vi "RPL_top_level_GUI_2.vi"() -> ()   [LabVIEW 2021]
uses:
  <vilib>/Utility/file.llb/Read Delimited Spreadsheet (string).vi
panel:
  out "Abort Status":string
  out "sol2":bool[](array[boolean])
  in  "Time Target (s)":dbl=1.0
  out "Array":string[][](array[string])
  in  "?":bool
  in  "Absolute Change":dbl
  out "ABORT\nACTIVATED":bool
  out "% Change":dbl[](array[numeric])
  in  "% Change":dbl
  out "all rows":string[][](array[string])
  in  "Fire Button":bool
  out "IGNITION":bool
  out "DEADMAN\nSWITCH":bool
  in  "Arm Button":bool
  out "POWER DISCONNECTED":bool
  in  "?":bool
  in  "SV6":bool
  in  "SV5":bool
  in  "SV4":bool
  in  "?":bool
  in  "SV3":bool
  in  "SV2":bool
  in  "SV1":bool
  in  "SV0":bool
  in  "GUITabs":T1(tab) caption="Tab Control"
  in  "Deadman Switch Pin":u16(ring) items=["FIO0", "FIO1", "FIO2", "FIO3", "FIO4", "FIO5", "FIO6", "FIO7", "EIO0", "EIO1", "EIO2", "EIO3", "EIO4", "EIO5", "EIO6", "EIO7", "CIO0", "CIO1", "CIO2", "CIO3", "MIO0", "MIO1", "MIO2"]
  in  "Solenoid Supply Pin":u16=5
  in  "LabJack Supply Pin":u16=7
  in  "Relay Supply Pin":u16=9
  in  "Igniter Pin":u16(ring)=7 items=["FIO0", "FIO1", "FIO2", "FIO3", "FIO4", "FIO5", "FIO6", "FIO7", "EIO0", "EIO1", "EIO2", "EIO3", "EIO4", "EIO5", "EIO6", "EIO7", "CIO0", "CIO1", "CIO2", "CIO3", "MIO0", "MIO1", "MIO2"]
  in  "LabJack IP Address":string="192.168.1.199"
  in  "LabJack Connection Type":u16(ring) items=["USB", "Ethernet"]
  in  "S: NO/NC":bool=TRUE
  in  "SV0 Pin":u16(ring)=8 items=["FIO0", "FIO1", "FIO2", "FIO3", "FIO4", "FIO5", "FIO6", "FIO7", "EIO0", "EIO1", "EIO2", "EIO3", "EIO4", "EIO5", "EIO6", "EIO7", "CIO0", "CIO1", "CIO2", "CIO3", "MIO0", "MIO1", "MIO2"]
  in  "SV1 Pin":u16(ring)=9 items=["FIO0", "FIO1", "FIO2", "FIO3", "FIO4", "FIO5", "FIO6", "FIO7", "EIO0", "EIO1", "EIO2", "EIO3", "EIO4", "EIO5", "EIO6", "EIO7", "CIO0", "CIO1", "CIO2", "CIO3", "MIO0", "MIO1", "MIO2"]
  in  "SV3 Pin":u16(ring)=11 items=["FIO0", "FIO1", "FIO2", "FIO3", "FIO4", "FIO5", "FIO6", "FIO7", "EIO0", "EIO1", "EIO2", "EIO3", "EIO4", "EIO5", "EIO6", "EIO7", "CIO0", "CIO1", "CIO2", "CIO3", "MIO0", "MIO1", "MIO2"]
  in  "SV2 Pin":u16(ring)=10 items=["FIO0", "FIO1", "FIO2", "FIO3", "FIO4", "FIO5", "FIO6", "FIO7", "EIO0", "EIO1", "EIO2", "EIO3", "EIO4", "EIO5", "EIO6", "EIO7", "CIO0", "CIO1", "CIO2", "CIO3", "MIO0", "MIO1", "MIO2"]
  in  "SV6 Pin":u16(ring)=14 items=["FIO0", "FIO1", "FIO2", "FIO3", "FIO4", "FIO5", "FIO6", "FIO7", "EIO0", "EIO1", "EIO2", "EIO3", "EIO4", "EIO5", "EIO6", "EIO7", "CIO0", "CIO1", "CIO2", "CIO3", "MIO0", "MIO1", "MIO2"]
  in  "SV5 Pin":u16(ring)=13 items=["FIO0", "FIO1", "FIO2", "FIO3", "FIO4", "FIO5", "FIO6", "FIO7", "EIO0", "EIO1", "EIO2", "EIO3", "EIO4", "EIO5", "EIO6", "EIO7", "CIO0", "CIO1", "CIO2", "CIO3", "MIO0", "MIO1", "MIO2"]
  in  "SV4 Pin":u16(ring)=12 items=["FIO0", "FIO1", "FIO2", "FIO3", "FIO4", "FIO5", "FIO6", "FIO7", "EIO0", "EIO1", "EIO2", "EIO3", "EIO4", "EIO5", "EIO6", "EIO7", "CIO0", "CIO1", "CIO2", "CIO3", "MIO0", "MIO1", "MIO2"]
  in  "S: NO/NC":bool=TRUE
  in  "S: NO/NC":bool=TRUE
  in  "S: NO/NC":bool=TRUE
  in  "S: NO/NC":bool=TRUE
  in  "S: NO/NC":bool=TRUE
  in  "S: NO/NC":bool=TRUE
  in  "R: NC/NO":bool=TRUE
  in  "R: NC/NO":bool=TRUE
  in  "R: NC/NO":bool=TRUE
  in  "R: NC/NO":bool=TRUE
  in  "R: NC/NO":bool=TRUE
  in  "R: NC/NO":bool=TRUE
  in  "R: NC/NO":bool=TRUE
  in  "TC1 Type":u16(ring)=7 items=["B", "E", "J", "K", "N", "R", "S", "T"]
  in  "TC2 Type":u16(ring)=3 items=["B", "E", "J", "K", "N", "R", "S", "T"]
  in  "TC1 +Channel":u16
  in  "TC2 -Channel":u16=3
  in  "TC2 +Channel":u16=2
  in  "TC1 -Channel":u16=1
  in  "PT2 Pin":u16=6
  in  "PT1 Pin":u16=8
  in  "PT3 Pin":u16=4
  in  "LP1 Pin":u16=10
  in  "k [N/m]":dbl=2000.0
  out "?":u32[](array[numeric])
  out "?":bool[](array[boolean])
  out "?":string[](array[string])
  in  "SV0":bool
  out "?":bool[](array[boolean])
  out "?":bool[](array[boolean])
  out "?":bool[](array[boolean])
  in  "SV1":bool
  in  "SV2":bool
  in  "SV3":bool
  out "?":bool[](array[boolean])
  in  "SV4":bool
  out "?":bool[](array[boolean])
  out "?":bool[](array[boolean])
  in  "SV5":bool
  in  "SV6":bool
  in  "Procedure Name":string
  in  "P#":u32
  in  "Add Procedure":bool
  in  "Remove Procedure":bool
  in  "Row":u32
  out "?":u32[](array[numeric])
  out "File Path":path[](array[path])
  out "?":bool
  out "?":bool
  out "?":bool
  out "?":bool
  out "?":bool
  out "?":bool
  out "?":bool
  out "?":bool
  out "?":bool
  out "?":bool
  out "?":bool
  out "?":bool
  out "?":bool
  in  "Dry Test-Run":bool
  out "LabJack Supply Voltage":dbl(slide) scale=0.0..5.0
  out "Solenoid Supply Voltage":dbl(slide) scale=0.0..14.0
  out "Relay Supply Voltage":dbl(slide) scale=0.0..5.0
  out "?":bool
  out "?":bool
  out "?":bool
  out "PT3: Chamber Pressure [psi]":dbl(knob) scale=0.0..500.0
  out "TC1: N2O Temp [°C]":dbl(slide) scale=-20.0..20.0
  out "TC2: Chamber Temp [°C]":dbl(slide) scale=-270.0..1260.0
  out "LP1: Thrust Reading [N]":dbl(slide) scale=0.0..250.0
  out "PT1: N2O Pressure [psi]":dbl(knob) scale=0.0..1000.0
  out "PT2: Ethanol Pressure [psi]":dbl(knob) scale=0.0..1000.0
  out "?":bool
  out "?":bool
  out "?":dbl[][](graph)
  in  "DATA LOGGING":bool
  in  "?":bool
  in  "?":bool
  # "SYSTEM FIRE OPERATION"
  # "CONTROL & ABORT STATUS"
  # "FEED SYSTEM SETTINGS"
  # "HIL TEST PARAMETERS"
  # "THERMOCOUPLE SETTINGS"
  # "SOLENOID VALVE & RELAY SETTINGS"
  # "CALIBRATION SETTINGS"
  # "POWER SYSTEM SETTINGS"
  # "THRUST MEASUREMENT SETTINGS"
  # "LINE & CHAMBER STATUS"
  # "RUNTANK FLOWRATE STATUS"
  # "DATA LOGGING"
  # "POWER SUPPLY STATUS"
  # "THRUST STATUS"
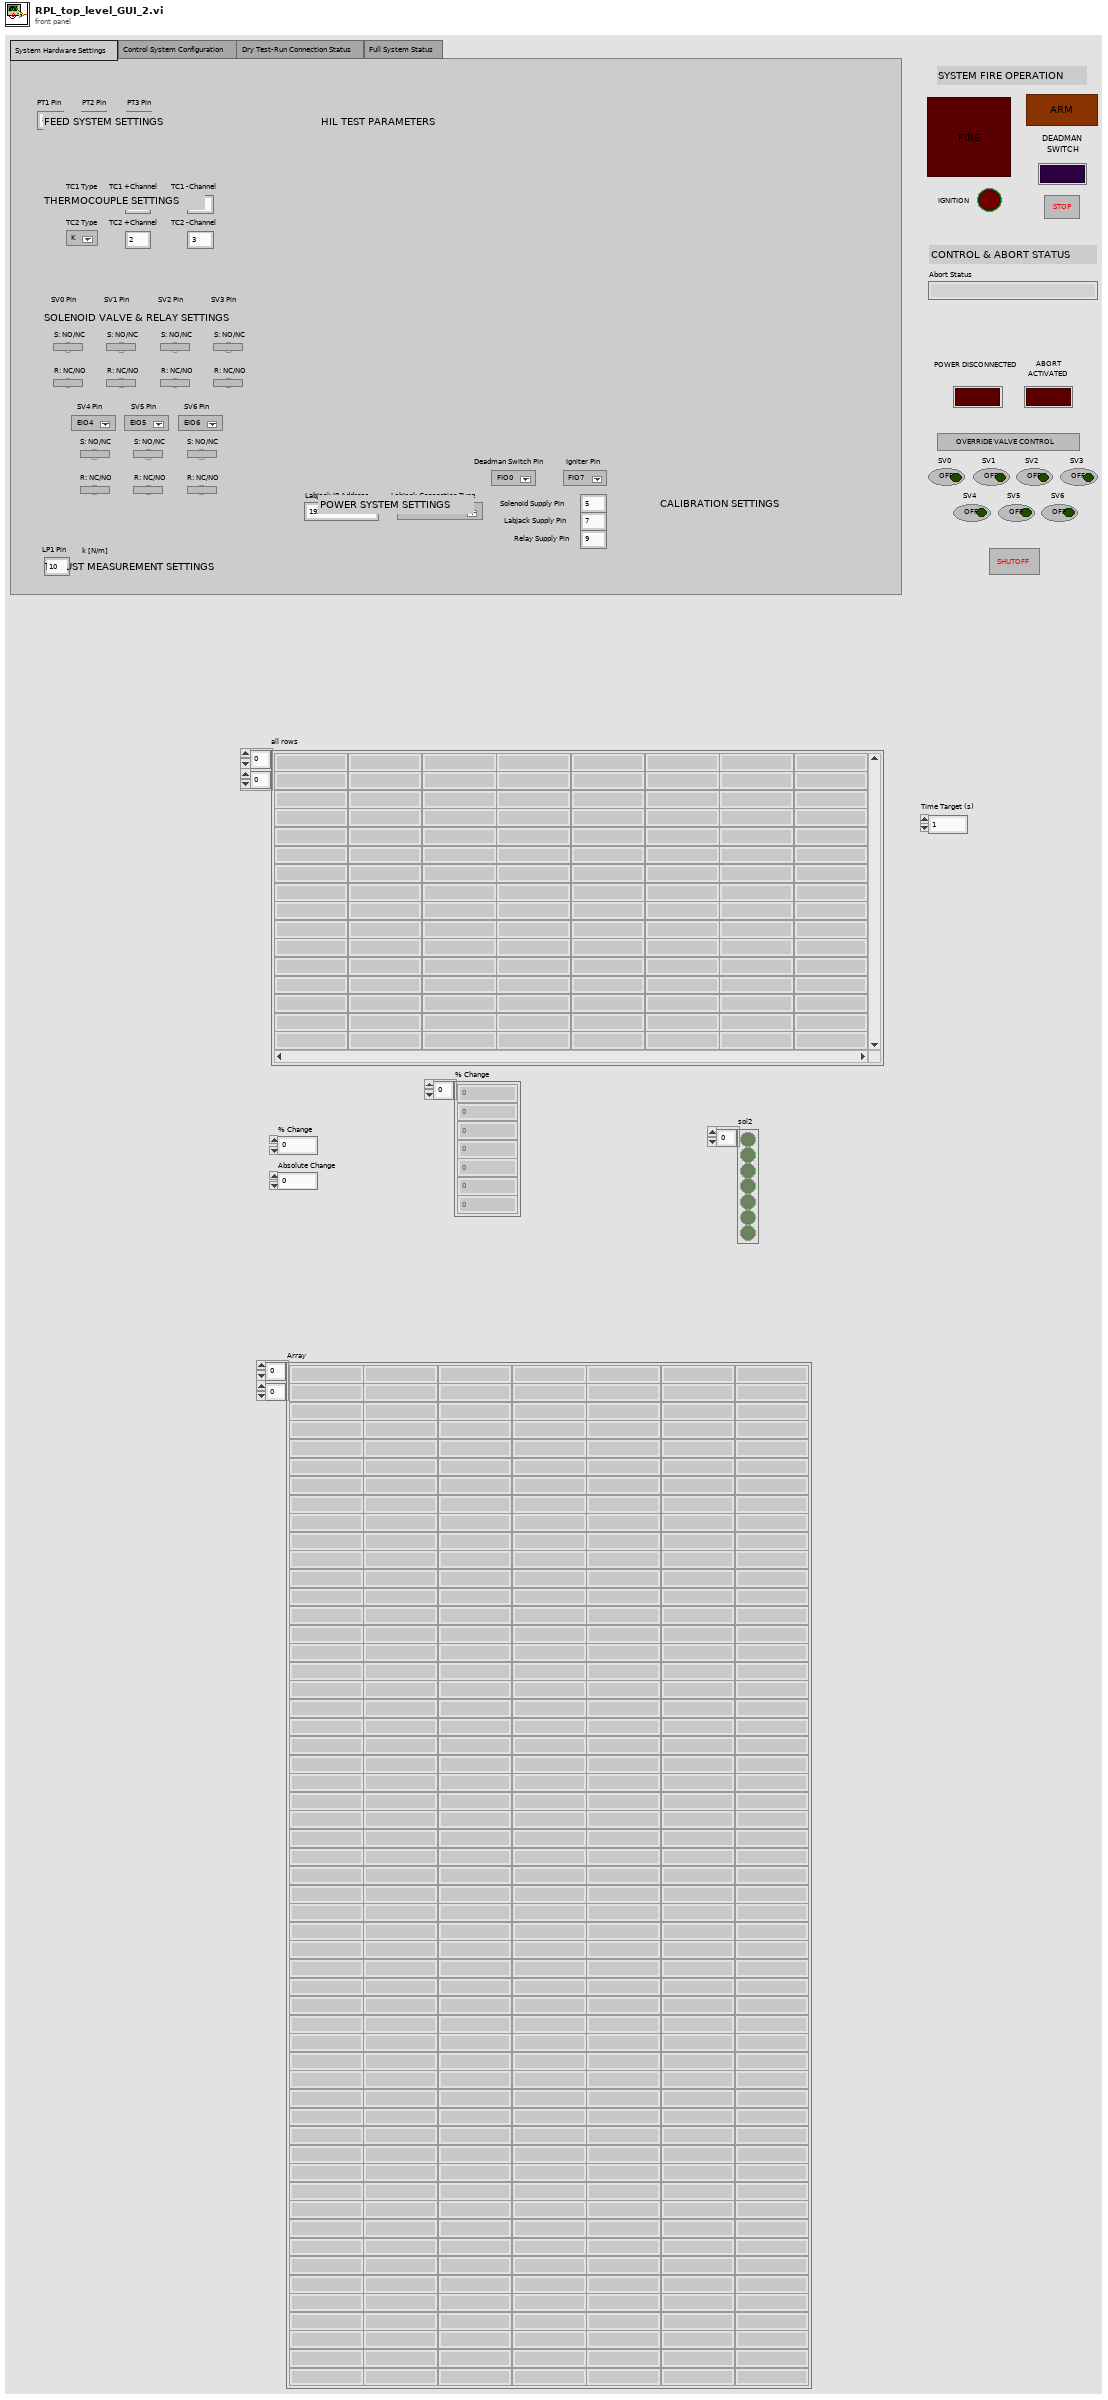
[diagram p1: front panel]
types:
  T1 = enum32{"System Hardware Settings", "Control System Configuration", "Dry Test-Run Connection Status", "Full System Status"}
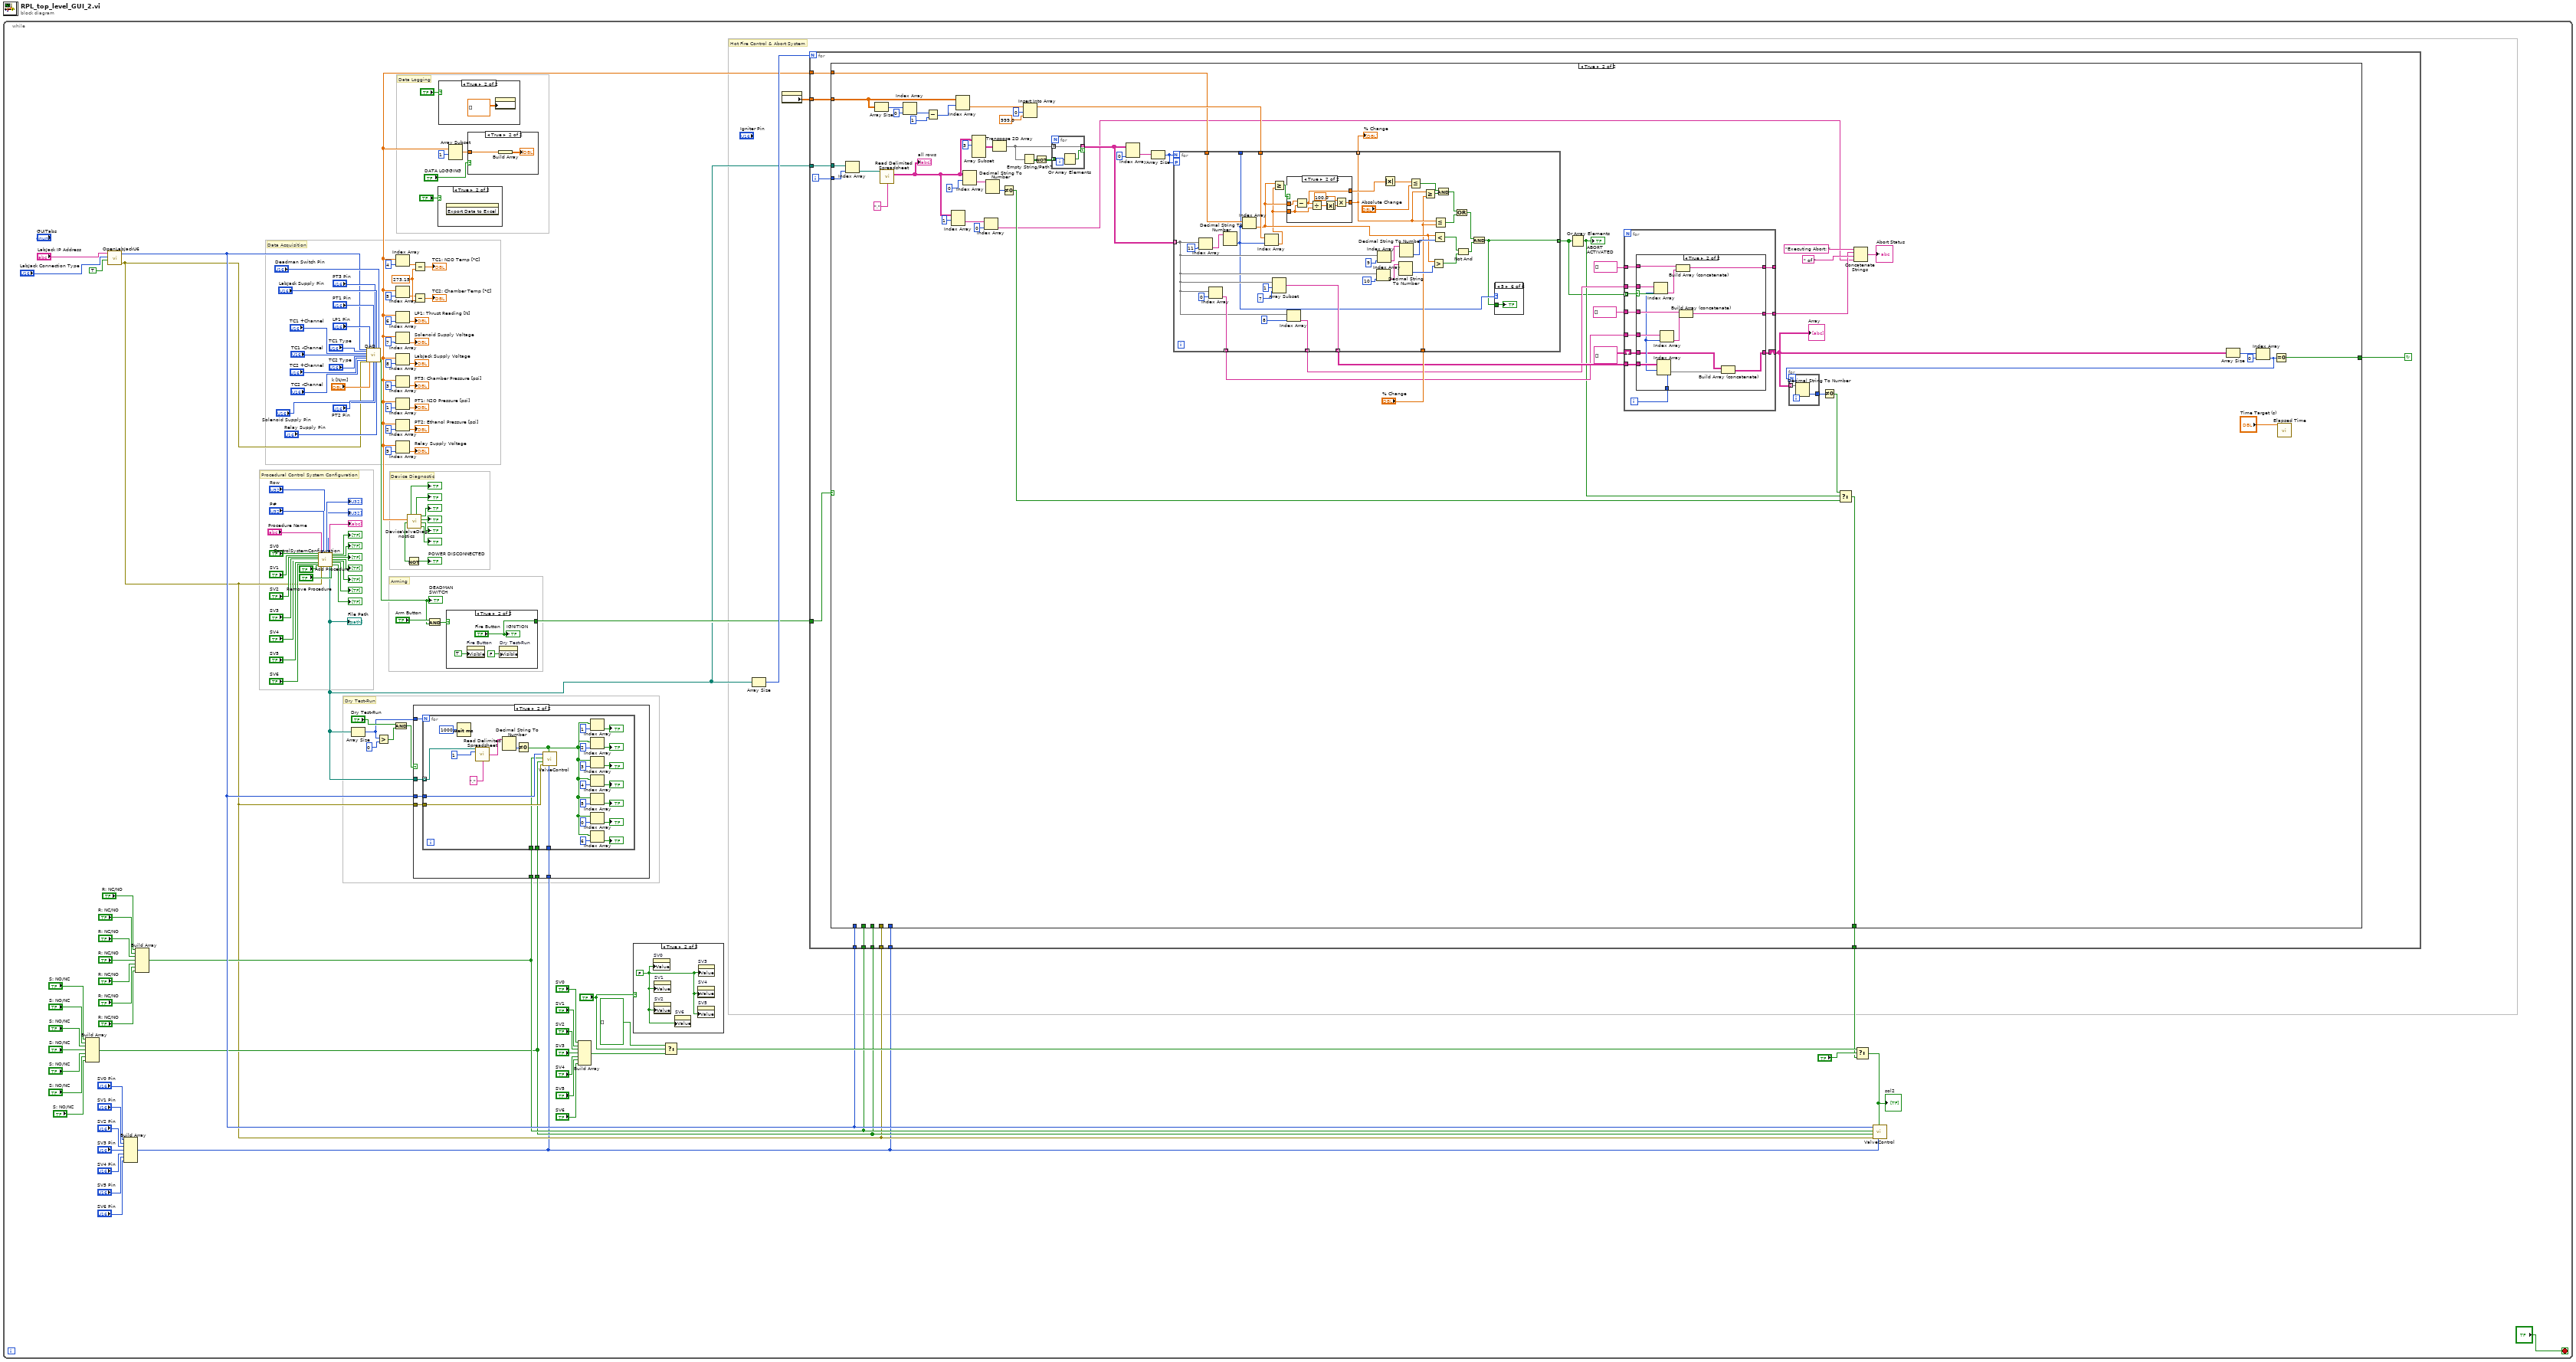
[diagram p0: block diagram]
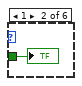
[diagram p5: hidden frame]
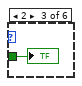
[diagram p6: hidden frame]
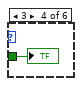
[diagram p7: hidden frame]
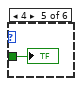
[diagram p8: hidden frame]
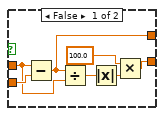
[diagram p9: hidden frame]
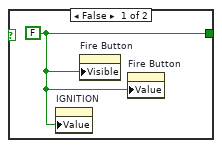
[diagram p12: hidden frame]
diagram:
  n1 = while {
    stop <- "?" stop-if-true
    w101 = 273.15 ("x")
    # "Hot Fire Control & Abort System"
    # "Dry Test-Run"
    # "Procedural Control System Configuration"
    # "Arming"
    # "Data Logging"
    # "Device Diagnostic"
    # "Data Acquisition"
    n2 = Build Array("S: NO/NC", "S: NO/NC", "S: NO/NC", "S: NO/NC", "S: NO/NC", "S: NO/NC", "S: NO/NC") -> (w9:bool[])
    n3 = call "OpenLabJackU6.vi"("Select First Found"=TRUE, "Connection Type"="LabJack Connection Type", "U6 Address"="LabJack IP Address") -> ("error out"=w8:errorcluster, "Handle"=w11:i32)  [unwired: 1 in, 1 out]
    n4 = Build Array("SV0 Pin", "SV1 Pin", "SV2 Pin", "SV3 Pin", "SV4 Pin", "SV5 Pin", "SV6 Pin") -> (w7:u16[])
    n5 = Build Array("R: NC/NO", "R: NC/NO", "R: NC/NO", "R: NC/NO", "R: NC/NO", "R: NC/NO", "R: NC/NO") -> (w10:bool[])
    n6 = call "ControlSystemConfiguration.vi"("SV0"="SV0", "SV1"="SV1", "SV2"="SV2", "SV3"="SV3", "SV4"="SV4", "SV5"="SV5", "SV6"="SV6", "Add Procedure"="Add Procedure", "Procedure Name"="Procedure Name", "error in"=w8, "P#"="P#", "Row"="Row", "Remove Procedure"="Remove Procedure") -> ("Row"=→"?":u32[], 16:→"?":u32[], 18:→"?":string[], "File Path"=w5:path[], 20:→"?":bool[], 21:→"?":bool[], 22:→"?":bool[], 23:→"?":bool[], 24:→"?":bool[], 25:→"?":bool[], 26:→"?":bool[])  [unwired: 3 in, 1 out]
    "File Path" <- w5
    n7 = Array Size(array=w5) -> (size(s)=w48:i32)
    n8 = call "DAQ.vi"("Handle In"=w11, "TC1 Type"="TC1 Type", "TC1 +Channel"="TC1 +Channel", "TC1 -Channel"="TC1 -Channel", "TC2 Type"="TC2 Type", "TC2 +Channel"="TC2 +Channel", "TC2 -Channel"="TC2 -Channel", "error in"=w8, "LP1 Pin"="LP1 Pin", "k [N/m]"="k [N/m]", "PT1 Pin"="PT1 Pin", "PT2 Pin"="PT2 Pin", "PT3 Pin"="PT3 Pin", "Solenoid Supply Pin"="Solenoid Supply Pin", "LabJack Supply Pin"="LabJack Supply Pin", "Relay Supply Pin"="Relay Supply Pin", "Deadman Switch Pin"="Deadman Switch Pin") -> ("Sensor Values"=w6:dbl[], "Deadman Switch"=w3:bool)  [unwired: 8 in, 1 out]
    "DEADMAN\nSWITCH" <- w3
    n9 = Greater?(x=w48, y=0) -> (0:w50:bool)
    n10 = And(x="Dry Test-Run", y=w50) -> (x .and. y?=w49:bool)
    n11 = Index Array(array=w6, index=4) -> (element=w100:dbl)
    n12 = Index Array(array=w6, index=5) -> (element=w99:dbl)
    n13 = Index Array(array=w6, index=6) -> (element=→"LP1: Thrust Reading [N]":dbl)
    n14 = Index Array(array=w6, index=7) -> (element=→"Solenoid Supply Voltage":dbl)
    n15 = Index Array(array=w6, index=8) -> (element=→"LabJack Supply Voltage":dbl)
    n16 = Index Array(array=w6, index=3) -> (element=→"PT3: Chamber Pressure [psi]":dbl)
    n17 = Index Array(array=w6, index=1) -> (element=→"PT1: N2O Pressure [psi]":dbl)
    n18 = Index Array(array=w6, index=2) -> (element=→"PT2: Ethanol Pressure [psi]":dbl)
    n19 = Index Array(array=w6, index=9) -> (element=→"Relay Supply Voltage":dbl)
    n20 = call "DeviceValveDiagnostics.vi"("Sensor Values"=w6) -> (0:→"?":bool, "Power Connected"=w82:bool, 4:→"?":bool, 6:→"?":bool, 7:→"?":bool, 8:→"?":bool, 9:→"?":bool)  [unwired: 2 out]
    n21 = Not(x=w82) -> (.not. x?=→"POWER DISCONNECTED":bool)
    n22 = Subtract(x=w100, y=w101) -> (x-y=→"TC1: N2O Temp [°C]":dbl)
    n23 = Subtract(x=w99, y=w101) -> (x-y=→"TC2: Chamber Temp [°C]":dbl)
    n24 = case shown="True" w49 {
      tunnel: w5 -> [_ w291]
      tunnel: w48 -> [_ w290]
      tunnel: w11 -> [_ w289]
      tunnel: w8 -> [_ w288]
      tunnel: w10 -> [_ w287]
      tunnel: w9 -> [_ w286]
      tunnel: w7 -> [_ w285]
      frame False {
      }
      frame True {
        n25 = for {
          N: w290 -> [_]
          tunnel: w291 -> [w315] mode=indexing
          tunnel: w289 -> [w304]
          tunnel: w288 -> [w303]
          tunnel: w287 -> [w301]
          tunnel: w286 -> [w300]
          tunnel: w285 -> [w299]
          n26 = Wait (ms)(milliseconds to wait=u32 1000) -> ()  [unwired: 1 out]
          n27 = call-poly <vilib>:"Read Delimited Spreadsheet.vi"("file path (dialog if empty)"=w315, "number of rows (all:-1)"=1, "delimiter (\\t)"="," ("delimiter (\\t)")) -> ("first row"=w313:string[])  [unwired: 7 in, 5 out]
          n28 = Decimal String To Number(string=w313) -> (number=w314:i32[])  [unwired: 2 in, 1 out]
          n29 = Not Equal To 0?(x=w314) -> (x != 0?=w305:bool[])
          n30 = call "ValveControl.vi"("SV Pin"=w299, "Solenoid States"=w305, "error in"=w303, "Solenoid NC/NO"=w300, "Relay NO/NC"=w301, "Handle In"=w304) -> ()  [unwired: 1 out]
          n31 = Index Array(array=w305, index=1) -> (element=→"?":bool)
          n32 = Index Array(array=w305, index=2) -> (element=→"?":bool)
          n33 = Index Array(array=w305, index=3) -> (element=→"?":bool)
          n34 = Index Array(array=w305, index=4) -> (element=→"?":bool)
          n35 = Index Array(array=w305, index=5) -> (element=→"?":bool)
          n36 = Index Array(array=w305, index=0) -> (element=→"?":bool)
          n37 = Index Array(array=w305, index=6) -> (element=→"?":bool)
        }
      }
    }
    n38 = Compound Arithmetic op=AND("Arm Button", w3) -> (w75:bool)
    n39 = case shown="True" "?" {
      frame False {
      }
      frame True {
        n40 = invoke class="WFChart (strict)" method="Export Data to Excel"() -> ()  [unwired: 3 in, 3 out]
      }
    }
    n41 = case shown="True" "?" {
      frame False {
      }
      frame True {
        n42 = property class="WFChart (strict)"("History Data"=dbl[][] []) -> ()  [unwired: 2 in, 2 out]
      }
    }
    n43 = case shown="True" w75 {
      tunnel: [w318 "Fire Button"] -> w13
      frame False {
        w318 = FALSE ("Visible")
        n44 = property on="IGNITION" class="Bool (strict)"("Value"=w318) -> ()  [unwired: 2 in, 2 out]
        n45 = property on="Fire Button" class="Bool (strict)"("Visible"=w318) -> ()  [unwired: 2 in, 2 out]
        n46 = property on="Fire Button" class="Bool (strict)"("Value"=w318) -> ()  [unwired: 2 in, 2 out]
      }
      frame True {
        n47 = property on="Fire Button" class="Bool (strict)"("Visible"=TRUE) -> ()  [unwired: 2 in, 2 out]
        n48 = property on="Dry Test-Run" class="Bool (strict)"("Visible"=FALSE) -> ()  [unwired: 2 in, 2 out]
        "IGNITION" <- "Fire Button"
      }
    }
    n49 = Array Subset(array=w6, index=1) -> (w79:dbl[])  [unwired: 1 in]
    n50 = case shown="True" "DATA LOGGING" {
      tunnel: w79 -> [_ w323]
      frame False {
      }
      frame True {
        n51 = Build Array(w323) -> (→"?":dbl[][])
      }
    }
    n52 = Build Array("SV0", "SV1", "SV2", "SV3", "SV4", "SV5", "SV6") -> (w18:bool[])
    n53 = case shown="True" "?" {
      frame False {
      }
      frame True {
        w284 = FALSE ("SV0")
        n54 = property on="SV0" class="Bool (strict)"("Value"=w284) -> ()  [unwired: 2 in, 2 out]
        n55 = property on="SV1" class="Bool (strict)"("Value"=w284) -> ()  [unwired: 2 in, 2 out]
        n56 = property on="SV2" class="Bool (strict)"("Value"=w284) -> ()  [unwired: 2 in, 2 out]
        n57 = property on="SV6" class="Bool (strict)"("Value"=w284) -> ()  [unwired: 2 in, 2 out]
        n58 = property on="SV4" class="Bool (strict)"("Value"=w284) -> ()  [unwired: 2 in, 2 out]
        n59 = property on="SV5" class="Bool (strict)"("Value"=w284) -> ()  [unwired: 2 in, 2 out]
        n60 = property on="SV3" class="Bool (strict)"("Value"=w284) -> ()  [unwired: 2 in, 2 out]
      }
    }
    n61 = Select(t=bool[] [], s="?", f=w18) -> (s? t:f=w15:bool[])
    n62 = Array Size(array=w5) -> (size(s)=w14:i32)
    n63 = property class="WFChart (strict)"() -> ("History Data"=w12:dbl[][])  [unwired: 2 in, 2 out]
    n64 = for {
      N: w14 -> [_]
      tunnel: w13 -> [w140]
      tunnel: w5 -> [w139]
      tunnel: w12 -> [w137]
      tunnel: w11 -> [w136]
      tunnel: w10 -> [w135]
      tunnel: w9 -> [w134]
      tunnel: w8 -> [w133]
      tunnel: w7 -> [w132]
      tunnel: w6 -> [w131]
      tunnel: [w130] -> w2
      i -> [w138]
      stop <- w129 continue-if-true
      n65 = case shown="True" w140 {
        tunnel: w139 -> [_ w188]
        tunnel: w138 -> [_ w187]
        tunnel: w137 -> [_ w177]
        tunnel: w136 -> [_ _]
        tunnel: w135 -> [_ _]
        tunnel: w134 -> [_ _]
        tunnel: w133 -> [_ _]
        tunnel: w132 -> [_ _]
        tunnel: w131 -> [_ w171]
        tunnel: [_ w151] -> w129
        tunnel: [_ w153] -> w130
        frame False {
        }
        frame True {
          n66 = Index Array(array=w188, index=w187) -> (element=w186:path)
          n67 = Array Size(array=w177) -> (size(s)=w183:i32[])
          n68 = call-poly <vilib>:"Read Delimited Spreadsheet.vi"("file path (dialog if empty)"=w186, "delimiter (\\t)"="," ("delimiter (\\t)")) -> ("all rows"=w144:string[][])  [unwired: 8 in, 5 out]
          "all rows" <- w144
          n69 = Index Array(array=w183, index=0) -> (element=w184:i32)
          n70 = Subtract(x=w184, y=1) -> (x-y=w185:i32)
          n71 = Index Array(array=w144, index (row)=1 ("index")) -> (element=w143:string[])  [unwired: 1 in]
          n72 = Index Array(array=w177, index (row)=w185) -> (element=w182:dbl[])  [unwired: 1 in]
          n73 = Index Array(array=w144, index (row)=0) -> (element=w149:string[])  [unwired: 1 in]
          n74 = Array Subset(array=w144, index (row)=3 ("index")) -> (w195:string[][])  [unwired: 3 in]
          n75 = Index Array(array=w143, index=0) -> (element=w141:string)
          n76 = Decimal String To Number(string=w149) -> (number=w189:i32[])  [unwired: 2 in, 1 out]
          n77 = Transpose 2D Array(2D array=w195) -> (transposed array=w193:string[][])
          n78 = Not Equal To 0?(x=w189) -> (x != 0?=w155:bool[])
          n79 = Empty String/Path?(string/path=w193) -> (empty?=w194:bool[][])
          n80 = Insert Into Array(array=w182, index=0, new element=999.0 ("new element/subarray")) -> (w172:dbl[])
          n81 = Not(x=w194) -> (.not. x?=w192:bool[][])
          n82 = for {
            tunnel: w193 -> [w282] mode=indexing
            tunnel: w192 -> [w283] mode=indexing
            tunnel: [w282] -> w173 mode=indexing if=w281
            n83 = Or Array Elements(Boolean array=w283) -> (logical OR=w281:bool)
          }
          n84 = Index Array(array=w173, index (col)=0 ("disabled index (col)")) -> (element=w176:string[])  [unwired: 1 in]
          n85 = Array Size(array=w176) -> (size(s)=w174:i32)
          n86 = for {
            N: w174 -> [_]
            tunnel: w173 -> [w246] mode=indexing
            tunnel: w171 -> [w259]
            tunnel: w172 -> [w258]
            tunnel: "% Change" -> [w231]
            workers-P: w174 -> [_]
            tunnel: [w232] -> w170 mode=indexing
            tunnel: [w226] -> w152 mode=indexing
            tunnel: [w248] -> w164 mode=indexing
            tunnel: [w245] -> w163 mode=indexing
            tunnel: [w244] -> w165 mode=indexing
            tunnel: [w227] -> _
            n87 = Index Array(array=w246, index=11) -> (element=w260:string)
            n88 = Index Array(array=w246, index=0) -> (element=w248:string)
            n89 = Decimal String To Number(string=w260) -> (number=w227:i32)  [unwired: 2 in, 1 out]
            n90 = Index Array(array=w259, index=w227) -> (element=w239:dbl)
            n91 = Index Array(array=w258, index=w227) -> (element=w238:dbl)
            n92 = Greater Or Equal?(x=w239, y=w238) -> (x >= y?=w240:bool)
            n93 = Array Subset(array=w246, index=1, length=7) -> (w244:string[])
            n94 = Index Array(array=w246, index=8) -> (element=w245:string)
            n95 = case shown="True" w240 {
              tunnel: w239 -> [w269 w280]
              tunnel: w238 -> [w270 w279]
              tunnel: [w268 w275] -> w232
              tunnel: [w267 w274] -> w235
              frame False {
                n96 = Subtract(x=w269, y=w270) -> (x-y=w267:dbl)
                n97 = Divide(x=w267, y=w269) -> (x/y=w273:dbl)
                n98 = Absolute Value(x=w273) -> (abs(x)=w272:dbl)
                n99 = Multiply(x=100.0, y=w272) -> (x*y=w268:dbl)
              }
              frame True {
                n100 = Subtract(x=w280, y=w279) -> (x-y=w274:dbl)
                n101 = Divide(x=w274, y=w279) -> (x/y=w278:dbl)
                n102 = Absolute Value(x=w278) -> (abs(x)=w277:dbl)
                n103 = Multiply(x=100.0, y=w277) -> (x*y=w275:dbl)
              }
            }
            n104 = Index Array(array=w246, index=10) -> (element=w254:string)
            n105 = Index Array(array=w246, index=9) -> (element=w256:string)
            n106 = Absolute Value(x=w235) -> (abs(x)=w229:dbl)
            n107 = Decimal String To Number(string=w254) -> (number=w252:i32)  [unwired: 2 in, 1 out]
            n108 = Decimal String To Number(string=w256) -> (number=w253:i32)  [unwired: 2 in, 1 out]
            n109 = Less Or Equal?(x=w229, y="Absolute Change") -> (x <= y?=w234:bool)
            n110 = Greater Or Equal?(x=w232, y=w231) -> (x >= y?=w233:bool)
            n111 = Greater?(x=w239, y=w252) -> (0:w242:bool)
            n112 = Less?(x=w239, y=w253) -> (x < y?=w243:bool)
            n113 = Less Or Equal?(x=w232, y=w231) -> (x <= y?=w237:bool)
            n114 = And(x=w234, y=w233) -> (x .and. y?=w230:bool)
            n115 = Or(x=w230, y=w237) -> (x .or. y?=w236:bool)
            n116 = Not And(1:w242, 2:w243) -> (0:w241:bool)
            n117 = And(x=w236, y=w241) -> (x .and. y?=w226:bool)
            n118 = case shown="5" w227 {
              tunnel: w226 -> [_ w262 w263 w264 w265 w266]
              frame 0, Default {
              }
              frame 1 {
                "?" <- w262
              }
              frame 2 {
                "?" <- w263
              }
              frame 3 {
                "?" <- w264
              }
              frame 4 {
                "?" <- w265
              }
              frame 5 {
                "?" <- w266
              }
            }
          }
          "% Change" <- w170
          n119 = Or Array Elements(Boolean array=w152) -> (logical OR=w154:bool)
          "ABORT\nACTIVATED" <- w154
          n120 = for {
            tunnel: w152 -> [w200] mode=indexing
            tunnel: w163 -> [w208]
            tunnel: w164 -> [w207]
            tunnel: w165 -> [w202]
            tunnel: string[] [] ("sorted array") -> [w203]
            tunnel: [w204] -> w146
            tunnel: string[] [] ("sorted array") -> [w205]
            tunnel: [w206] -> _
            shift-right: [w201] -> w158
            shift-left: string[][] [] -> [w199]
            i -> [w209]
            n121 = case shown="True" w200 {
              tunnel: w205 -> [w212 w225]
              tunnel: w209 -> [_ w216]
              tunnel: w208 -> [_ w224]
              tunnel: w203 -> [w211 w222]
              tunnel: w207 -> [_ w221]
              tunnel: [w212 w219] -> w206
              tunnel: [w211 w218] -> w204
              tunnel: w202 -> [_ w217]
              tunnel: [w210 w213] -> w201
              tunnel: w199 -> [w210 w215]
              frame False {
              }
              frame True {
                n122 = Index Array(array=w224, index=w216) -> (element=w220:string)
                n123 = Index Array(array=w217, index (row)=w216) -> (element=w214:string[])  [unwired: 1 in]
                n124 = Index Array(array=w221, index=w216) -> (element=w223:string)
                n125 = Build Array (concatenate)(w225, w220) -> (w219:string[])
                n126 = Build Array (concatenate)(w222, w223) -> (w218:string[])
                n127 = Build Array (concatenate)(w215, w214) -> (w213:string[][])
              }
            }
          }
          "Array" <- w158
          n128 = Concatenate Strings("Executing Abort: " ("string"), w146, " of " ("string"), w141) -> (→"Abort Status":string)
          n129 = Array Size(array=w158) -> (size(s)=w161:i32[])
          n130 = Index Array(array=w161, index=0) -> (element=w159:i32)
          n131 = for {
            N: w159 -> [_]
            tunnel: w158 -> [w197] mode=indexing
            tunnel: [w198] -> w157
            n132 = Decimal String To Number(string=w197) -> (number=w198:i32[])  [unwired: 2 in, 1 out]
          }
          n133 = Not Equal To 0?(x=w157) -> (x != 0?=w156:bool[])
          n134 = Select(t=w156, s=w154, f=w155) -> (s? t:f=w153:bool[])
          n135 = Equal To 0?(x=w159) -> (x = 0?=w151:bool)
          n136 = call "Elapsed Time"("Time Target (s)"="Time Target (s)") -> ()  [unwired: 11 in, 8 out]
        }
      }
    }
    n137 = Select(t=w15, s="?", f=w2) -> (s? t:f=w1:bool[])
    "sol2" <- w1
    n138 = call "ValveControl.vi"("SV Pin"=w7, "Solenoid States"=w1, "error in"=w8, "Solenoid NC/NO"=w9, "Relay NO/NC"=w10, "Handle In"=w11) -> ()  [unwired: 1 out]
  }
